vi "Autonomous Independent.vi"   [LabVIEW 2016]
doc: "This VI is called when autonomous begins, and will automatically be terminated when autonomous ends. You can carry out timed or sensor driven robot movement independently without needing to return to the caller."
uses:
  <vilib>/Rock Robotics/WPI/Solenoid/WPI_SolenoidValue.ctl
  <vilib>/Rock Robotics/Network Tables/NT Read String.vi
  <vilib>/Rock Robotics/WPI/Solenoid/WPI_SolenoidSetEnum.vi
types:
  T1 = typedef "WPI_SolenoidValue.ctl" = enum16{"Off", "On", "Forward", "Reverse"}
  T2 = cluster{"RobotDrive":string, "Gyro":string, "Mtr 1":string, "Mtr 2":string}
  T3 = typedef "WPI_GyroDevRef.ctl" = cluster{"DevStatus":errorcluster, "Analog Channel":T4, "Offset":dbl, "Gain (VoltsPerDegree/Second)":dbl, "Gyro Type":enum16{"Analog", "XRS450"}, "Handle":i32, "SPI Bus":T5, "Device Found":bool, "Sample Rate":dbl, "Calibrate On Open":bool}
  T4 = typedef "FPGA_AIChannel.ctl" = enum8{"AI 0", "AI 1", "AI 2", "AI 3", "AI MXP 0", "AI MXP 1", "AI MXP 2", "AI MXP 3", "Invalid"}
  T5 = typedef "spi_bus.ctl" = enum16{"SPI On-Board, CS0", "SPI On-Board, CS1", "SPI On-Board, CS2", "SPI On-Board, CS3", "SPI MXP", "Invalid"}
  T6 = typedef "WPI_SolenoidDevRef.ctl" = cluster{"DevStatus":errorcluster, "Pneumatics Control Module":u8, "Forward Solenoid Channel":T7, "Reverse Solenoid Channel":T7}
  T7 = typedef "WPI_SolenoidChannel.ctl" = enum8{"Solenoid 0", "Solenoid 1", "Solenoid 2", "Solenoid 3", "Solenoid 4", "Solenoid 5", "Solenoid 6", "Solenoid 7", "Invalid"}
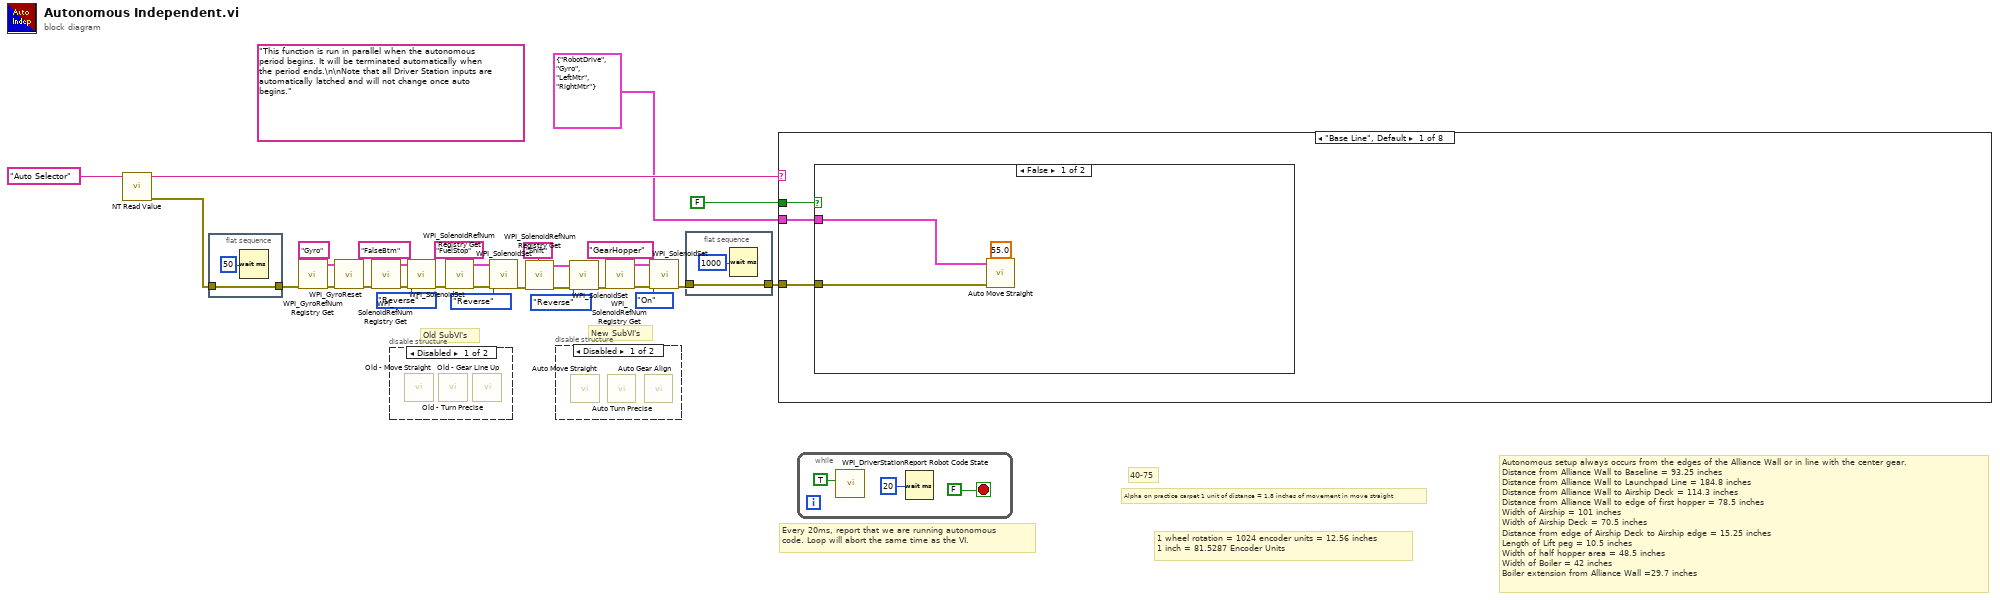
[diagram p0: block diagram]
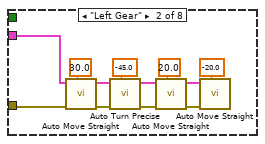
[diagram p5: hidden frame]
diagram:
  (unwired) "This function is run in parallel when the autonomous period begins. It will be terminated automatically when the period ends.\n\nNote that all Driver Station inputs are automatically latched and will not change once auto begins."
  # "40-75"
  # "Alpha on practice carpet 1 unit of distance = 1.8 inches of movement in move straight"
  # "New SubVI's"
  # "Old SubVI's"
  # "Autonomous setup always occurs from the edges of the Alliance Wall or in line with the center gear.\nDistance from Alliance Wall to Baseline = 93.25 inches\nDistance from Alliance Wall to Launchpad Line = 184.8 inches\nDistance from Alliance Wall to Airship Deck = 114.3 inches\nDistance from Alliance Wall to edge of first hopper = 78.5 inches\nWidth of Airship = 101 inches\nWidth of Airship Deck = 70.5 inches\nDistance from edge of Airship Deck to Airship edge = 15.25 inches\nLength of Lift peg = 10.5 inches\nWidth of half hopper area = 48.5 inches\nWidth of Boiler = 42 inches\nBoiler extension from Alliance Wall =29.7 inches"
  # "1 wheel rotation = 1024 encoder units = 12.56 inches\n1 inch = 81.5287 Encoder Units"
  # "Every 20ms, report that we are running autonomous\ncode. Loop will abort the same time as the VI."
  n1 = call-poly <vilib>:"NT Read Value.vi"("Name"="Auto Selector") -> ("error out"=w29:errorcluster, "String"=w30:string)  [unwired: 9 in]
  n2 = flat-sequence {
    tunnel: [w32] -> w26
    tunnel: w29 -> [w32]
    frame #0 {
      n3 = Wait (ms)(milliseconds to wait=u32 50) -> ()  [unwired: 1 out]
    }
  }
  n4 = call <vilib>:"WPI_GyroRefNum Registry Get.vi"("error in (no error)"=w26, "refnum name"="Gyro") -> ("error out"=w25:errorcluster, "GyroDevRef"=w24:T3)  [unwired: 8 in]
  n5 = call <vilib>:"WPI_GyroReset.vi"("error in"=w25, "GyroDevRef"=w24) -> ("error out"=w7:errorcluster)  [unwired: 8 in, 1 out]
  n6 = call <vilib>:"WPI_SolenoidRefNum Registry Get.vi"("error in (no error)"=w7, "refnum name"="FalseBtm") -> ("error out"=w17:errorcluster, "SolenoidDevRef"=w16:T6)  [unwired: 8 in]
  n7 = disable-structure shown="Disabled" {
    frame Disabled {
      n8 = call "Old - Move Straight.vi"() -> ()  [unwired: 11 in, 1 out]
      n9 = call "Old - Turn Precise.vi"() -> ()  [unwired: 11 in, 1 out]
      n10 = call "Old - Gear Line Up.vi"() -> ()  [unwired: 11 in, 1 out]
    }
    frame Enabled {
    }
  }
  n11 = call-poly <vilib>:"WPI_SolenoidSet.vi"("error in (no error)"=w17, "Value"=WPI_SolenoidValue."Reverse", "SolenoidDevRef"=w16) -> ("error out"=w11:errorcluster)  [unwired: 7 in, 1 out]
  n12 = call <vilib>:"WPI_SolenoidRefNum Registry Get.vi"("error in (no error)"=w11, "refnum name"="FuelStop") -> ("error out"=w14:errorcluster, "SolenoidDevRef"=w13:T6)  [unwired: 8 in]
  n13 = call-poly <vilib>:"WPI_SolenoidSet.vi"("error in (no error)"=w14, "Value"=WPI_SolenoidValue."Reverse", "SolenoidDevRef"=w13) -> ("error out"=w1:errorcluster)  [unwired: 7 in, 1 out]
  n14 = call <vilib>:"WPI_SolenoidRefNum Registry Get.vi"("error in (no error)"=w1, "refnum name"="Shift") -> ("error out"=w6:errorcluster, "SolenoidDevRef"=w5:T6)  [unwired: 8 in]
  n15 = disable-structure shown="Disabled" {
    frame Disabled {
      n16 = call "Auto Move Straight.vi"() -> ()  [unwired: 10 in, 2 out]
      n17 = call "Auto Turn Precise.vi"() -> ()  [unwired: 10 in, 2 out]
      n18 = call "Auto Gear Align.vi"() -> ()  [unwired: 10 in, 2 out]
    }
    frame Enabled {
    }
  }
  n19 = call-poly <vilib>:"WPI_SolenoidSet.vi"("error in (no error)"=w6, "Value"=WPI_SolenoidValue."Reverse", "SolenoidDevRef"=w5) -> ("error out"=w2:errorcluster)  [unwired: 7 in, 1 out]
  n20 = call <vilib>:"WPI_SolenoidRefNum Registry Get.vi"("error in (no error)"=w2, "refnum name"="GearHopper") -> ("error out"=w22:errorcluster, "SolenoidDevRef"=w21:T6)  [unwired: 8 in]
  n21 = call-poly <vilib>:"WPI_SolenoidSet.vi"("error in (no error)"=w22, "Value"=WPI_SolenoidValue."On", "SolenoidDevRef"=w21) -> ("error out"=w18:errorcluster)  [unwired: 7 in, 1 out]
  n22 = flat-sequence {
    tunnel: [w34] -> w8
    tunnel: w18 -> [w34]
    frame #0 {
      n23 = Wait (ms)(milliseconds to wait=u32 1000) -> ()  [unwired: 1 out]
    }
  }
  n24 = case shown="\"Base Line\", Default" w30 {
    tunnel: FALSE ("No Sensors") -> [w38 _ _ _ _ _ _ _]
    tunnel: T2 {"RobotDrive"="RobotDrive", "Gyro"="Gyro", "Mtr 1"="LeftMtr", "Mtr 2"="RightMtr"} ("Refnum's") -> [w37 w48 _ _ _ _ _ _]
    tunnel: w8 -> [w36 w49 _ _ _ _ _ _]
    frame "Base Line", Default {
      n25 = case shown="False" w38 {
        tunnel: w37 -> [w41 _]
        tunnel: w36 -> [w39 _]
        frame False {
          n26 = call "Auto Move Straight.vi"("Target Distance"=55.0, "Error In"=w39, "Refnum's In"=w41) -> ()  [unwired: 7 in, 2 out]
        }
        frame True {
        }
      }
    }
    frame "Left Gear" {
      n27 = call "Auto Move Straight.vi"("Target Distance"=30.0, "Error In"=w49, "Refnum's In"=w48) -> ("Error Out"=w53:errorcluster, "Refnum's Out"=w52:T2)  [unwired: 7 in]
      n28 = call "Auto Turn Precise.vi"("Target Distance"=-45.0, "Error In"=w53, "Refnum's In"=w52) -> ("Error Out"=w51:errorcluster, "Refnum's Out"=w50:T2)  [unwired: 7 in]
      n29 = call "Auto Move Straight.vi"("Target Distance"=20.0, "Error In"=w51, "Refnum's In"=w50) -> ("Error Out"=w43:errorcluster, "Refnum's Out"=w42:T2)  [unwired: 7 in]
      n30 = call "Auto Move Straight.vi"("Target Distance"=-20.0, "Error In"=w43, "Refnum's In"=w42) -> ()  [unwired: 7 in, 2 out]
    }
    frame "Center Gear" {
    }
    frame "Right Gear" {
    }
    frame "Left Gear with Boiler" {
    }
    frame "Left Gear with Hopper" {
    }
    frame "Right Gear with Boiler" {
    }
    frame "Right Gear with Hopper" {
    }
  }
  n31 = while {
    stop <- FALSE stop-if-true
    n32 = call <vilib>:"WPI_DriverStationReport Robot Code State.vi"("Autonomous"=TRUE) -> ()  [unwired: 10 in, 1 out]
    n33 = Wait (ms)(milliseconds to wait=u32 20) -> ()  [unwired: 1 out]
  }
